vi "Format numeric command string.vi"(5 "Number":dbl, 7 "Command":string) -> (1 "String":string)   [LabVIEW 2015]
doc: "Concatenates a command string and a number to form a numerical command for the Harvard pump.\n\nModified from original which is Copyright 2005, National Instruments Corporation.\n\nModifications Copyright 2009, Jeff Gelles, Brandeis University"
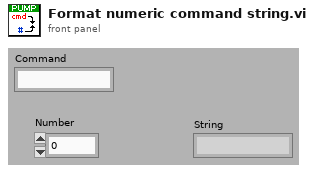
[diagram p1: front panel]
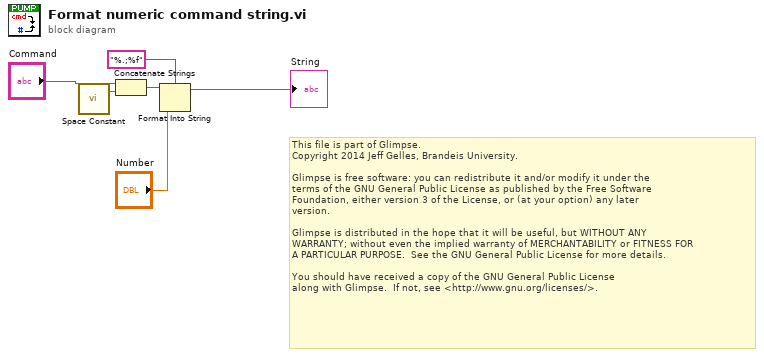
[diagram p0: block diagram]
diagram:
  # "This file is part of Glimpse. \nCopyright 2014 Jeff Gelles, Brandeis University.    \n\nGlimpse is free software: you can redistribute it and/or modify it under the \nterms of the GNU General Public License as published by the Free Software \nFoundation, either version 3 of the License, or (at your option) any later \nversion.\n\nGlimpse is distributed in the hope that it will be useful, but WITHOUT ANY \nWARRANTY; without even the implied warranty of MERCHANTABILITY or FITNESS FOR \nA PARTICULAR PURPOSE.  See the GNU General Public License for more details.\n\nYou should have received a copy of the GNU General Public License\nalong with Glimpse.  If not, see <http://www.gnu.org/licenses/>."
  n1 = call <vilib>:"Space Constant.vi"() -> ("String"=w1:string)
  n2 = Concatenate Strings("Command", w1) -> (w3:string)
  n3 = Format Into String(format string="%.;%f", initial string=w3, "Number") -> (resulting string=→"String":string)  [unwired: 1 in, 1 out]
